vi "calc_conveyor_2.vi"(10 "Conveyor Command Inputs":T5, 11 "ConveyorV2 Inputs":T4) -> (3 "Conveyor Outputs":T1)   [LabVIEW 2012]
uses:
  Input_Command_Conveyor.ctl
  Sensor_Input_ConveyorV2.ctl
  Conveyor_outputsV2.ctl
  3-Ball-Conveyor_Module_State.ctl
  T_Roller module state.ctl
panel:
  out "Shot Ball":bool
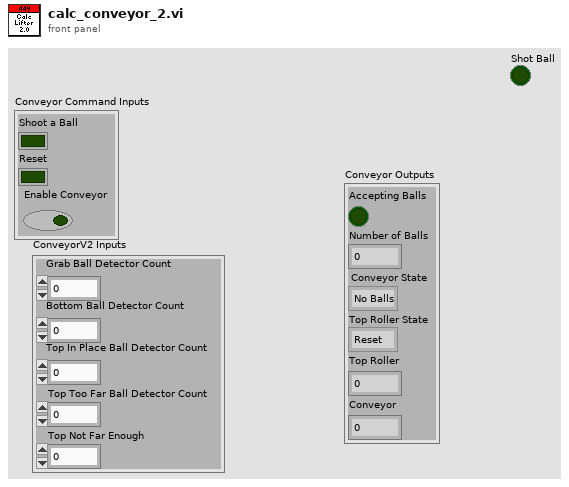
[diagram p1: front panel]
types:
  T1 = typedef "Conveyor_outputsV2.ctl" = cluster{"Accepting Balls":bool, "Number of Balls":i32, "Conveyor State":T2, "Top Roller State":T3, "Top Roller":dbl, "Conveyor":dbl}
  T2 = typedef "3-Ball-Conveyor_Module_State.ctl" = enum16{"No Balls", "Collecting Ball", "Holding 1", "Pushing Ball Out", "Holding 2", "Lowering Ball", "Reset", "Disabled"}
  T3 = typedef "T_Roller module state.ctl" = enum16{"Reset", "Disabled", "Waiting for Ball", "Holding", "Ball not far enough", "Ball too far", "Firing"}
  T4 = typedef "Sensor_Input_ConveyorV2.ctl" = cluster{"Grab Ball Detector Count":i32, "Bottom Ball Detector Count":i32, "Top In Place Ball Detector Count":i32, "Top Too Far Ball Detector Count":i32, "Top Not Far Enough":i32}
  T5 = typedef "Input_Command_Conveyor.ctl" = cluster{"Shoot a Ball":bool, "Reset":bool, "Enable Conveyor":bool}
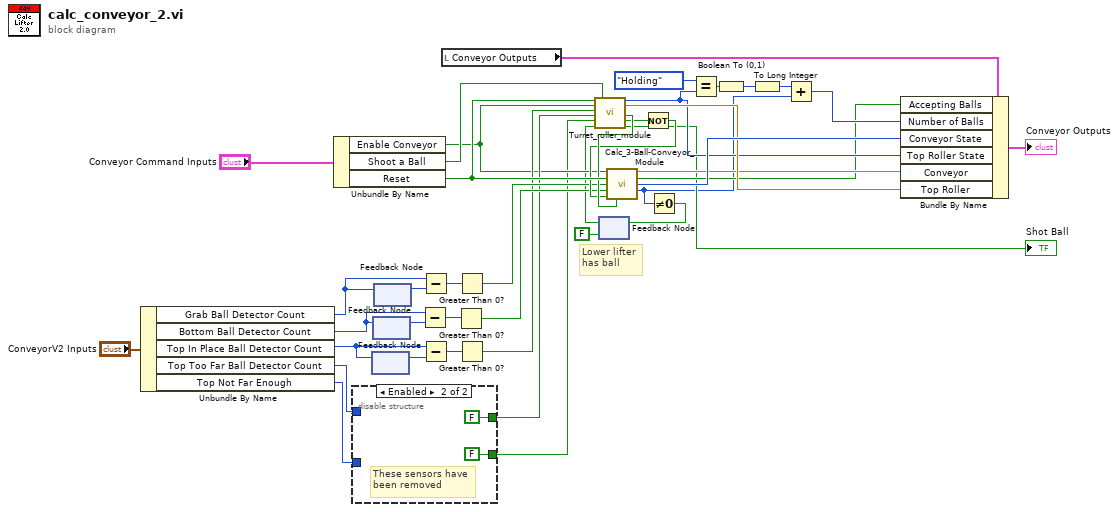
[diagram p0: block diagram]
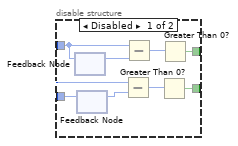
[diagram p2: hidden frame]
diagram:
  # "Lower lifter\nhas ball"
  n1 = Unbundle By Name("ConveyorV2 Inputs") -> ("Grab Ball Detector Count"=w20:i32, "Bottom Ball Detector Count"=w16:i32, "Top In Place Ball Detector Count"=w4:i32, "Top Too Far Ball Detector Count"=w2:i32, "Top Not Far Enough"=w1:i32)
  n2 = Unbundle By Name("Conveyor Command Inputs") -> ("Enable Conveyor"=w10:bool, "Shoot a Ball"=w40:bool, "Reset"=w39:bool)
  n3 = disable-structure shown="Enabled" {
    disable-tunnel: [w48 FALSE ("Ball too far")] -> w11
    disable-tunnel: [w46 FALSE ("Ball not far enough")] -> w5
    disable-tunnel: w2 -> [w45 _]
    disable-tunnel: w1 -> [w42 _]
    frame Disabled {
      n4 = feedback #1() -> (w44:i32)  [unwired: 1 in]
      n5 = feedback-in #1(w45) -> ()
      n6 = feedback #2() -> (w43:i32)  [unwired: 1 in]
      n7 = feedback-in #2(w42) -> ()
      n8 = Subtract(x=w42, y=w43) -> (x-y=w47:i32)
      n9 = Subtract(x=w45, y=w44) -> (x-y=w49:i32)
      n10 = Greater Than 0?(x=w47) -> (x > 0?=w46:bool)
      n11 = Greater Than 0?(x=w49) -> (x > 0?=w48:bool)
    }
    frame Enabled {
      # "These sensors have\nbeen removed"
    }
  }
  n12 = feedback #3() -> (w3:i32)  [unwired: 1 in]
  n13 = feedback-in #3(w4) -> ()
  n14 = feedback #4() -> (w17:i32)  [unwired: 1 in]
  n15 = feedback-in #4(w16) -> ()
  n16 = feedback-in #5(w20) -> ()
  n17 = feedback #5() -> (w21:i32)  [unwired: 1 in]
  n18 = Subtract(x=w16, y=w17) -> (x-y=w15:i32)
  n19 = Subtract(x=w20, y=w21) -> (x-y=w19:i32)
  n20 = Subtract(x=w4, y=w3) -> (x-y=w13:i32)
  n21 = local read "Conveyor Outputs"() -> (w34:T1)
  n22 = Greater Than 0?(x=w15) -> (x > 0?=w14:bool)
  n23 = Greater Than 0?(x=w19) -> (x > 0?=w18:bool)
  n24 = Greater Than 0?(x=w13) -> (x > 0?=w12:bool)
  n25 = feedback #6(FALSE) -> (w6:bool)
  n26 = call "Turret_roller_module.vi"("Reset"=w39, "Enable"=w10, "Ball Detected"=w12, "Ball too far"=w11, "Ball not far enough"=w5, "Lower Conveyor has Ball"=w6, "Shoot"=w40) -> ("Turret Roller State"=w28:T3, "T Roller Motor"=w31:dbl, "Acquired Ball"=w38:bool, "Accepting Balls"=w32:bool, "Shot Ball"=→"Shot Ball":bool)  [unwired: 8 in]
  n27 = Not(x=w32) -> (.not. x?=w37:bool)
  n28 = call "Calc_3-Ball-Conveyor_Module.vi"("Enable"=w10, "Reset"=w39, "Grab Sensor"=w18, "Bottom Sensor"=w14, "Ball in Turret"=w37, "Ball is out"=w38) -> ("Motor Speed"=w30:dbl, "Accepting Balls"=w23:bool, "State"=w33:T2, "Ball Count"=w9:i32)  [unwired: 6 in]
  n29 = Not Equal To 0?(x=w9) -> (x != 0?=w8:bool)
  n30 = feedback-in #6(w8) -> ()
  n31 = Equal?(x=T_Roller_module_state."Holding" ("Turret Roller State"), y=w28) -> (x = y?=w27:bool)
  n32 = Boolean To (0,1)(Boolean=w27) -> (0, 1=w26:i16)
  n33 = To Long Integer(number=w26) -> (32bit integer=w24:i32)
  n34 = Add(x=w24, y=w9) -> (x+y=w25:i32)
  n35 = Bundle By Name(cluster=w34, "Accepting Balls"=w23, "Number of Balls"=w25, "Conveyor State"=w33, "Top Roller State"=w28, "Conveyor"=w30, "Top Roller"=w31) -> (→"Conveyor Outputs":T1)
